vi "Unflatten Attr Priv.vi"(5 "Data Types Dict":variant, 6 "After First Tag String":string, 7 "Parsed Header":T1, 8 "error in":errorcluster, 10 "Parent ID (empty)":string, 11 "Tree Dict":variant) -> (0 "error out":errorcluster, 3 "Tree Dictionary Out":variant, 4 "After First Tag String":string)   [LabVIEW 2020, in "NI_VIAnCFGDataStructure.lvlib" / "Tree.lvclass"]
uses:
  <vilib>/addons/analyzer/VIAnCFGDataStructure/Tree Manager/Tree.lvclass
  <vilib>/addons/analyzer/VIAnCFGDataStructure/Tree Manager/Private/Parsed Header.ctl
  <vilib>/addons/analyzer/VIAnCFGDataStructure/Tree Data/Tree Data.lvclass
  <vilib>/Utility/error.llb/Error Cluster From Error Code.vi
  <vilib>/addons/analyzer/VIAnCFGDataStructure/Tree Manager/API/Generate Hash.vi
  <vilib>/ErrorRing/Error Ring.xnode
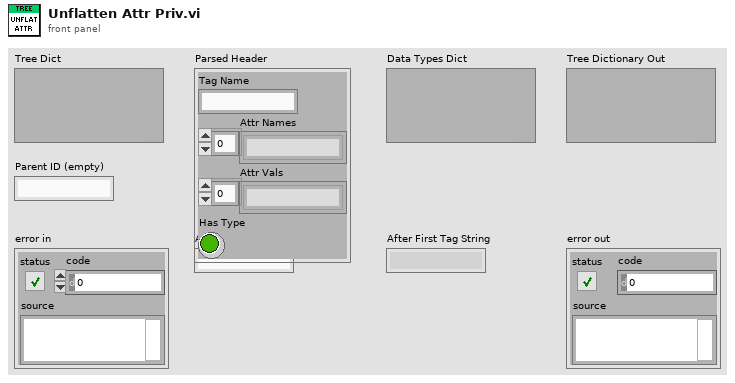
[diagram p1: front panel]
types:
  T1 = typedef "NI_VIAnCFGDataStructure.lvlib/Tree.lvclass/Parsed Header.ctl" = cluster{"Tag Name":string, "Attr Names":string[], "Attr Vals":string[], "Has Type":bool}
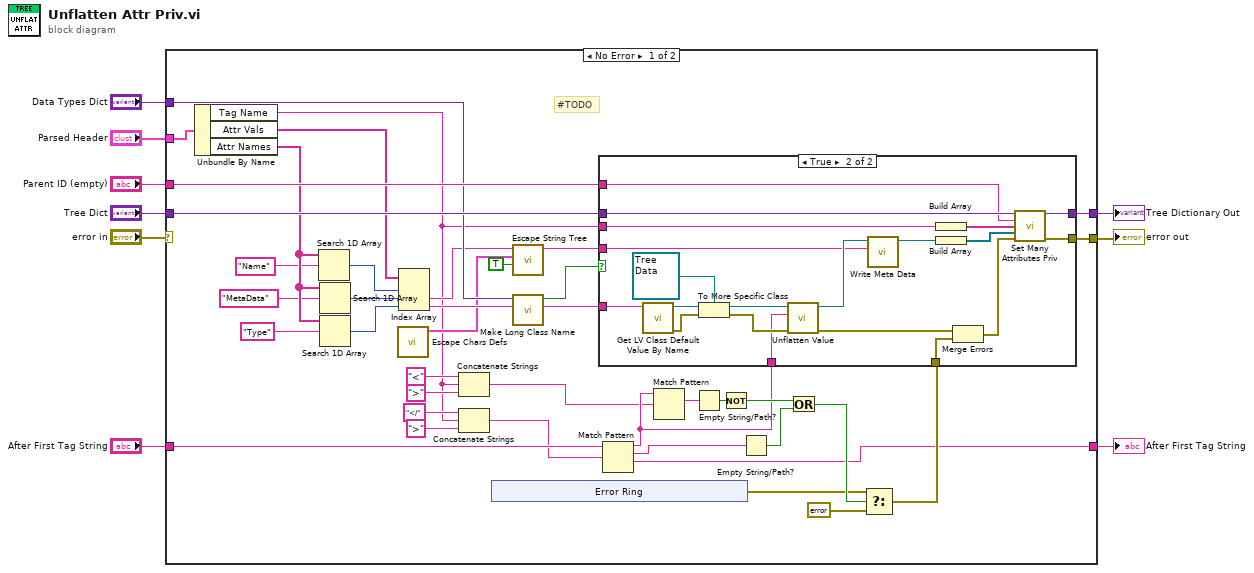
[diagram p0: block diagram]
diagram:
  n1 = case shown="No Error" "error in" {
    selector: "error in" -> [_ w79]
    tunnel: "Data Types Dict" -> [w22 _]
    tunnel: "Parent ID (empty)" -> [w46 _]
    tunnel: "Tree Dict" -> [w45 w78]
    tunnel: [w44 w79] -> w6
    tunnel: [w43 w78] -> w5
    tunnel: [w36 w77] -> w4
    tunnel: "After First Tag String" -> [w34 w77]
    tunnel: "Parsed Header" -> [w30 _]
    frame No Error {
      # "#TODO"
      n2 = Unbundle By Name(w30) -> ("Tag Name"=w12:string, "Attr Vals"=w32:string[], "Attr Names"=w31:string[])
      n3 = Search 1D Array(1D array=w31, element="Name") -> (index of element=w29:i32)  [unwired: 1 in]
      n4 = Search 1D Array(1D array=w31, element="MetaData") -> (index of element=w25:i32)  [unwired: 1 in]
      n5 = Search 1D Array(1D array=w31, element="Type") -> (index of element=w27:i32)  [unwired: 1 in]
      n6 = call <vilib>:"Escape Chars Defs.vi"() -> ("Escapes"=w18:cluster{"String":string, "Escape":string}[])  [unwired: 11 in]
      n7 = Index Array(array=w32, index #1=w29, index #2=w25, index #3=w27) -> (element #2=w20:string, element #3=w21:string)  [unwired: 1 out]
      n8 = Concatenate Strings("<" ("string"), w12, ">" ("string")) -> (w11:string)
      n9 = Concatenate Strings("</" ("string"), w12, ">" ("string")) -> (w10:string)
      n10 = xnode "Error Ring"() -> ("error out"=w33:errorcluster)
      n11 = call <vilib>:"Escape String Tree.vi"("Reverse? (False)"=TRUE, "Escapes"=w18, "String In"=w20) -> ("String Out"=w19:string)  [unwired: 8 in]
      n12 = call <vilib>:"Make Long Class Name.vi"("Short Class Name"=w21, "Data Types Dict"=w22) -> ("Long Class Name"=w23:string, "Found"=w48:bool)  [unwired: 8 in]
      n13 = Match Pattern(string=w34, regular expression=w10) -> (before substring=w37:string, match substring=w35:string, after substring=w36:string)  [unwired: 1 in, 1 out]
      n14 = Match Pattern(string=w37, regular expression=w11) -> (match substring=w38:string)  [unwired: 1 in, 3 out]
      n15 = Empty String/Path?(string/path=w38) -> (empty?=w39:bool)
      n16 = Not(x=w39) -> (.not. x?=w40:bool)
      n17 = Empty String/Path?(string/path=w35) -> (empty?=w41:bool)
      n18 = Or(x=w40, y=w41) -> (x .or. y?=w42:bool)
      n19 = Select(t=w33, s=w42, f=errorcluster {"status"=FALSE, "code"=0, "source"=""}) -> (s? t:f=w47:errorcluster)
      n20 = case shown="True" w48 {
        tunnel: w19 -> [_ w65]
        tunnel: w37 -> [_ w64]
        tunnel: [w50 w63] -> w43
        tunnel: [w51 w62] -> w44
        tunnel: w45 -> [w50 w61]
        tunnel: w46 -> [_ w60]
        tunnel: w12 -> [_ w59]
        tunnel: w47 -> [w51 w53]
        tunnel: w23 -> [_ w55]
        frame False {
        }
        frame True {
          n21 = call <vilib>:"Get LV Class Default Value By Name.vi"("class name"=w55) -> ("error out"=w68:errorcluster, "object"=w71:refnum<class>)  [unwired: 9 in]
          n22 = To More Specific Class(target class=refnum<class "Tree Data.lvclass"> refnum ("Tree Data In"), reference=w71, error in=w68) -> (specific class reference=w69:refnum<class "Tree Data.lvclass">, error out=w67:errorcluster)
          n23 = call-dynamic "Unflatten Value.vi"("Error In"=w67, "Value"=w64, "Tree Data In"=w69) -> ("Error Out"=w54:errorcluster, "Tree Data Out"=w66:refnum<class "Tree Data.lvclass">)  [unwired: 7 in]
          n24 = call <vilib>:"Write Meta Data.vi"("Meta Data"=w65, "Tree Data In"=w66) -> ("Tree Data Out"=w57:refnum<class "Tree Data.lvclass">)  [unwired: 9 in]
          n25 = Build Array(w59) -> (w58:string[])
          n26 = Build Array(w57) -> (w56:refnum<class "Tree Data.lvclass">[])
          n27 = Merge Errors(w54, w53) -> (w52:errorcluster)
          n28 = call <vilib>:"Set Many Attributes Priv.vi"("Tree Dictionary Out"=w61, "Unique ID"=w60, "Name"=w58, "Data"=w56, "error in"=w52) -> ("Tree Dictionary Out"=w63:variant, "error out"=w62:errorcluster)  [unwired: 8 in, 1 out]
        }
      }
    }
    frame Error {
    }
  }
  "error out" <- w6
  "Tree Dictionary Out" <- w5
  "After First Tag String" <- w4
